vi "Decoding Test Packet.vi"(8 "error in (no error)":errorcluster, 11 "Test Packet Input":T2) -> (0 "error out":errorcluster)   [LabVIEW 2013]
uses:
  source/Control Packets/ControlPacket/Control Packet Type -- enum.ctl
  source/Control Packets/ControlPacket/ControlPacket.lvclass
  <vilib>/addons/_JKI Toolkits/Caraya/classes/Test/Test.lvclass
  <vilib>/addons/_JKI Toolkits/Caraya/classes/Assert/Assert.lvclass
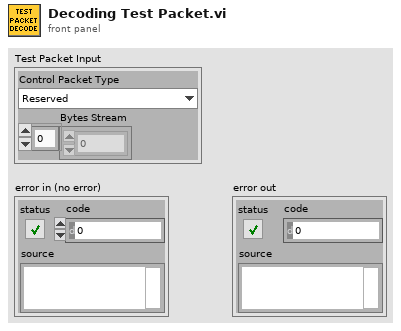
[diagram p1: front panel]
types:
  T1 = typedef "MQTT_Control_Packets.lvlib/ControlPacket.lvclass/Control Packet Type -- enum.ctl" = enum16{"Reserved", "CONNECT", "CONNACK", "PUBLISH", "PUBACK", "PUBREC", "PUBREL", "PUBCOMP", "SUBSCRIBE", "SUBACK", "UNSUBSCRIBE", "UNSUBACK", "PINGREQ", "PINGRESP", "DISCONNECT", "AUTH"}
  T2 = cluster{"Control Packet Type":T1, "Bytes Stream":u8[]}
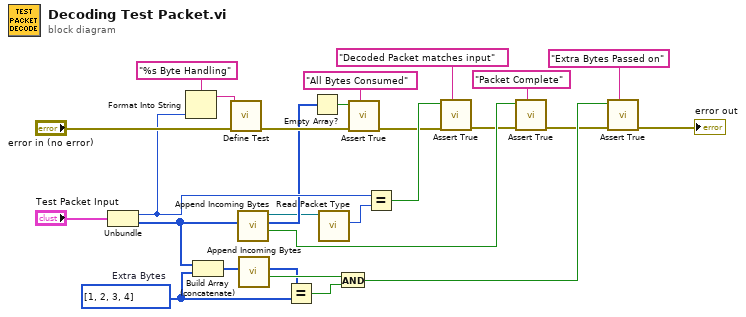
[diagram p0: block diagram]
diagram:
  w27 = u8[] [1, 2, 3, 4]  # Extra Bytes
  n1 = Unbundle("Test Packet Input") -> ("Control Packet Type"=w10:T1, "Bytes Stream"=w5:u8[])
  n2 = Format Into String(format string="%s Byte Handling", w10) -> (resulting string=w11:string)  [unwired: 2 in, 1 out]
  n3 = Build Array (concatenate)(w5, w27) -> (w6:u8[])
  n4 = call <vilib>:"Define Test.vi"("error in (no error)"="error in (no error)", "Label (VI Title)"=w11) -> ("error out"=w15:errorcluster)  [unwired: 9 in]
  n5 = call "Append Incoming Bytes.vi"("Incoming Packets"=w5) -> ("Complete Packet"=w21:bool, "Remaining Packets"=w2:u8[], "ControlPacket"=w1:refnum<class "ControlPacket.lvclass">)  [unwired: 7 in, 1 out]
  n6 = call "Append Incoming Bytes.vi"("Incoming Packets"=w6) -> ("Complete Packet"=w8:bool, "Remaining Packets"=w7:u8[])  [unwired: 7 in, 2 out]
  n7 = Equal?(x=w7, y=w27) -> (x = y?=w9:bool)
  n8 = Empty Array?(array=w2) -> (empty?=w16:bool)
  n9 = call "Read Packet Type.vi"("ControlPacket in"=w1) -> ("Control Packet Type"=w3:T1)  [unwired: 9 in, 1 out]
  n10 = And(x=w8, y=w9) -> (x .and. y?=w24:bool)
  n11 = call <vilib>:"Assert True.vi"("Label"="All Bytes Consumed" ("Label (VI Title)"), "error in (no error)"=w15, "True?"=w16) -> ("error out"=w17:errorcluster)  [unwired: 8 in]
  n12 = Equal?(x=w10, y=w3) -> (x = y?=w18:bool)
  n13 = call <vilib>:"Assert True.vi"("Label"="Decoded Packet matches input" ("Label (VI Title)"), "error in (no error)"=w17, "True?"=w18) -> ("error out"=w20:errorcluster)  [unwired: 8 in]
  n14 = call <vilib>:"Assert True.vi"("Label"="Packet Complete" ("Label (VI Title)"), "error in (no error)"=w20, "True?"=w21) -> ("error out"=w23:errorcluster)  [unwired: 8 in]
  n15 = call <vilib>:"Assert True.vi"("Label"="Extra Bytes Passed on" ("Label (VI Title)"), "error in (no error)"=w23, "True?"=w24) -> ("error out"=→"error out":errorcluster)  [unwired: 8 in]
